vi "filter folder list.vi"(7 "folder depth":i32=-1, 11 "All Folders":path[](array[path])) -> (3 "All Folders out":path[](array[path]), 5 "max length":i32)   [LabVIEW 2023]
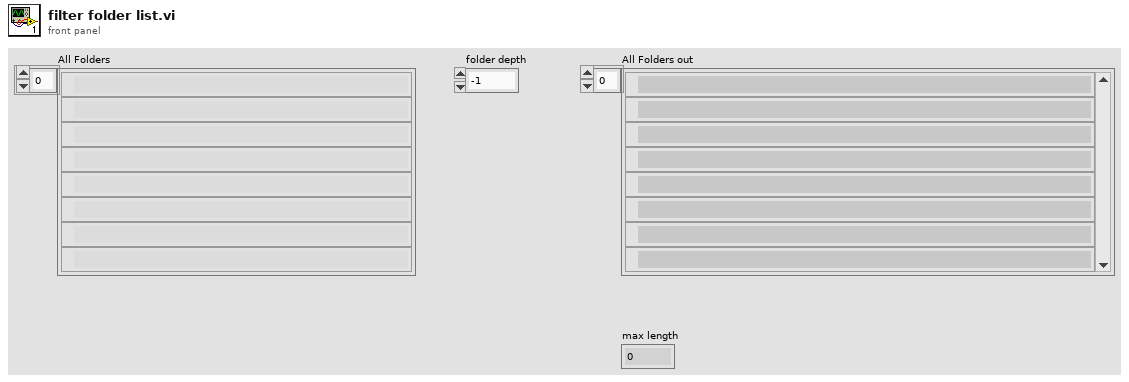
[diagram p1: front panel]
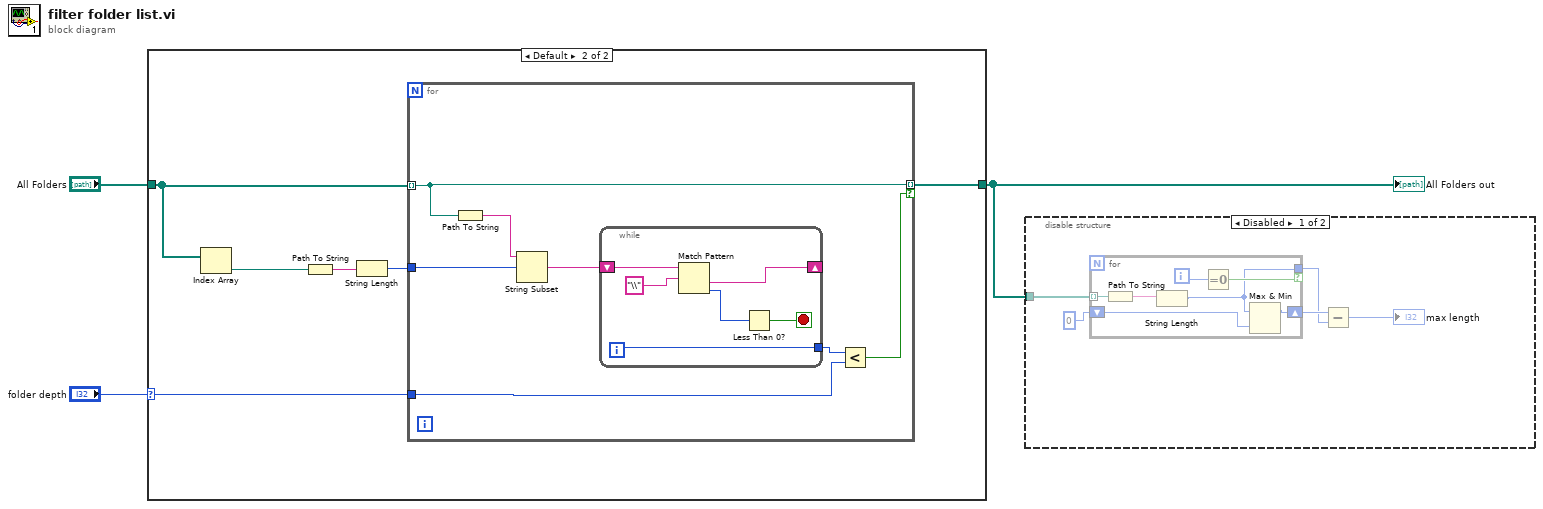
[diagram p0: block diagram]
diagram:
  n1 = case shown="Default" "folder depth" {
    selector: "folder depth" -> [_ w5]
    tunnel: "All Folders" -> [w4 w7]
    tunnel: [w4 w6] -> w1
    frame -1 {
    }
    frame Default {
      n2 = Index Array(array=w7) -> (element=w10:path)  [unwired: 1 in]
      n3 = Path To String(path=w10) -> (string=w9:string)
      n4 = String Length(string=w9) -> (length=w8:i32)
      n5 = for {
        tunnel: w7 -> [w15] mode=indexing
        tunnel: w8 -> [w16]
        tunnel: [w15] -> w6 mode=indexing if=w12
        tunnel: w5 -> [w13]
        n6 = Path To String(path=w15) -> (string=w17:string)
        n7 = String Subset(string=w17, offset (0)=w16) -> (substring=w11:string)  [unwired: 1 in]
        n8 = while {
          shift-right: [w22] -> _
          shift-left: w11 -> [w23]
          tunnel: [w19] -> w14
          i -> [w19]
          stop <- w20 stop-if-true
          n9 = Match Pattern(string=w23, regular expression="\\") -> (after substring=w22:string, offset past match=w21:i32)  [unwired: 1 in, 2 out]
          n10 = Less Than 0?(x=w21) -> (x < 0?=w20:bool)
        }
        n11 = Less?(x=w14, y=w13) -> (x < y?=w12:bool)
      }
    }
  }
  "All Folders out" <- w1
  n12 = disable-structure shown="Disabled" {
    disable-tunnel: w1 -> [w27 _]
    frame Disabled {
      n13 = for {
        tunnel: w27 -> [w35] mode=indexing
        tunnel: [w31] -> w25 if=w32
        shift-right: [w30] -> w26
        shift-left: 0 -> [w29]
        i -> [w33]
        n14 = Path To String(path=w35) -> (string=w34:string)
        n15 = String Length(string=w34) -> (length=w31:i32)
        n16 = Equal To 0?(x=w33) -> (x = 0?=w32:bool)
        n17 = Max & Min(x=w31, y=w29) -> (max(x,y)=w30:i32)  [unwired: 1 out]
      }
      n18 = Subtract(x=w26, y=w25) -> (x-y=→"max length":i32)
    }
    frame Enabled {
    }
  }
